vi "Array Variant to Array of Variants.vi"(8 "error in (no error)":errorcluster, 11 "Arrray Variant":variant) -> (0 "error out":errorcluster, 3 "[Variant]":variant[](array[variant]))   [LabVIEW 2018, in "TwinCAT ADS.lvclass"]
uses:
  TwinCAT ADS.lvclass
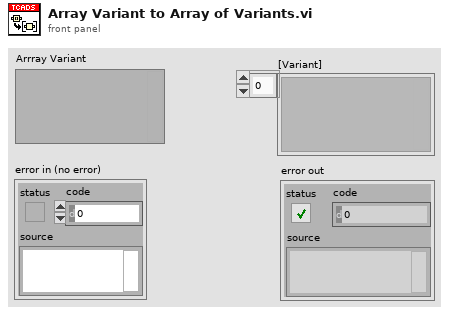
[diagram p1: front panel]
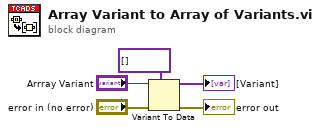
[diagram p0: block diagram]
diagram:
  n1 = Variant To Data(error in="error in (no error)", type=variant[] [] ("appended array"), Variant="Arrray Variant") -> (data=→"[Variant]":variant[], error out=→"error out":errorcluster)
